vi "Generic command handler.vi"(8 "error in (no error)":errorcluster, 10 "Message in":refnum<class "GenericMessage.lvclass">, 11 "StageSPIM in":refnum<class "StageSPIM.lvclass">) -> (0 "error out":errorcluster, 2 "value":string, 3 "StageSPIM out":refnum<class "StageSPIM.lvclass">)   [LabVIEW 2012, in "StageSPIM.lvclass"]
doc: "The generic_command_handler processes the command 'generic'. Commands which are not part of the predefined list of commands fall under the 'generic' command for special activity."
uses:
  StageSPIM.lvclass
  <vilib>/Distrio/Murmex/Murmex/Murmex.lvclass
  <vilib>/Distrio/Murmex/Message/Message.lvclass
  <vilib>/Distrio/Murmex/ProceedMessage/ProceedMessage.lvclass
  <vilib>/Distrio/Murmex/GenericMessage/GenericMessage.lvclass
panel:
  # "This method is called when the GENERIC\ntrigger is sent. \n\nOverride this method when your component needs to\nrespond to this trigger. \n\nCall parent for proper implementation"
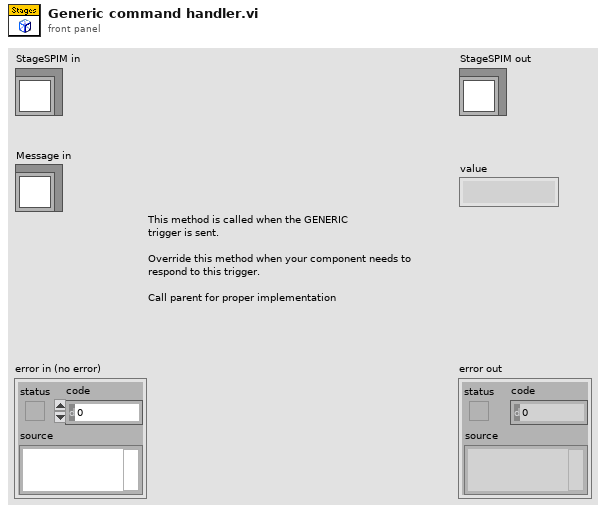
[diagram p1: front panel]
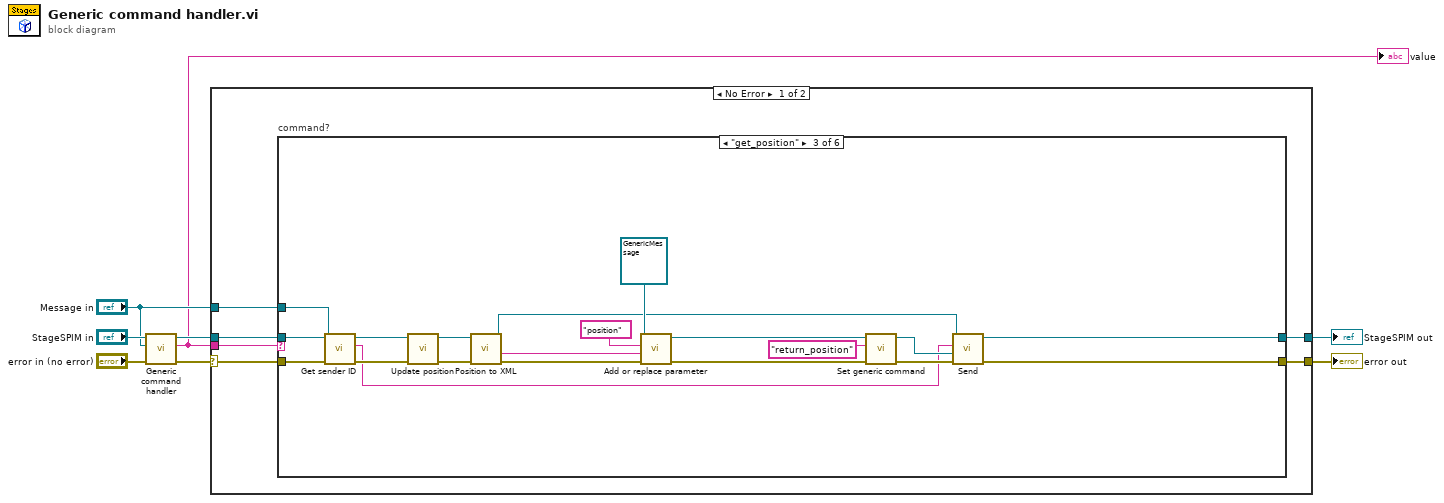
[diagram p0: block diagram]
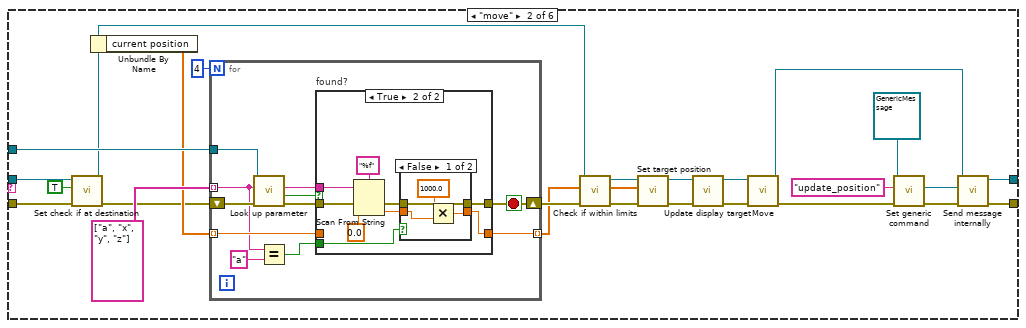
[diagram p3: hidden frame]
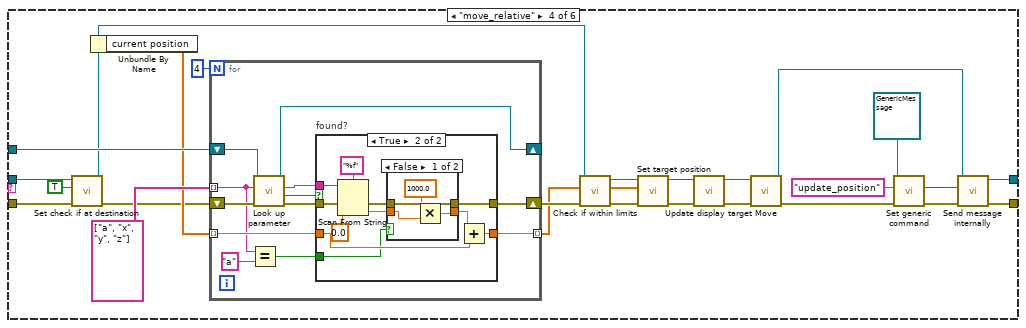
[diagram p6: hidden frame]
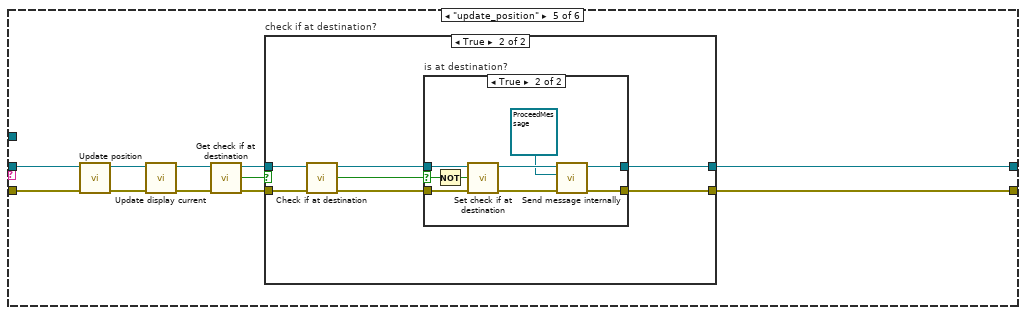
[diagram p9: hidden frame]
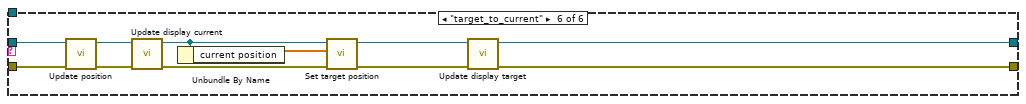
[diagram p12: hidden frame]
diagram:
  n1 = call-parent "Generic command handler.vi"("error in (no error)"="error in (no error)", "Message in"="Message in", "Murmex in"="StageSPIM in") -> ("error out"=w6:errorcluster, "value"=w3:string, "Murmex out"=w5:refnum<class "StageSPIM.lvclass">)  [unwired: 6 in]
  "value" <- w3
  n2 = case shown="No Error" w6 {
    selector: w6 -> [w13 w189]
    tunnel: w3 -> [w14 _]
    tunnel: w5 -> [w12 w190]
    tunnel: "Message in" -> [w11 _]
    tunnel: [w10 w189] -> w2
    tunnel: [w9 w190] -> w1
    frame No Error {
      n3 = case "command?" shown="\"get_position\"" w14 {
        tunnel: w13 -> [w15 w31 w89 w104 w157 w186]
        tunnel: w12 -> [w16 w33 w75 w106 w156 w185]
        tunnel: w11 -> [_ w38 w88 w111 _ _]
        tunnel: [w15 w24 w71 w97 w151 w180] -> w10
        tunnel: [w16 w21 w72 w94 w152 w178] -> w9
        frame Default {
        }
        frame "move" {
          n4 = call-dynamic "Set check if at destination.vi"("error in (no error)"=w31, "check if at destination"=TRUE, "StageSPIM in"=w33) -> ("error out"=w30:errorcluster, "StageSPIM out"=w32:refnum<class "StageSPIM.lvclass">)  [unwired: 7 in]
          n5 = Unbundle By Name(w32) -> ("current position"=w35:dbl[])
          n6 = for {
            N: 4 -> [_]
            shift-right: [w46] -> w39
            shift-left: w30 -> [w53]
            tunnel: string[] ["a", "x", "y", "z"] -> [w44] mode=indexing
            tunnel: w35 -> [w48] mode=indexing
            tunnel: [w47] -> w34 mode=indexing
            tunnel: w38 -> [w49]
            stop <- w46 stop-if-true
            n7 = call <vilib>:"Look up parameter.vi"("error in (no error)"=w53, "name"=w44, "Message in"=w49) -> ("error out"=w52:errorcluster, "found?"=w51:bool, "key"=w50:string)  [unwired: 5 in, 1 out]
            n8 = Equal?(x=w44, y="a") -> (x = y?=w43:bool)
            n9 = case "found?" shown="True" w51 {
              tunnel: w52 -> [w55 w64]
              tunnel: [w55 w59] -> w46
              tunnel: w50 -> [_ w62]
              tunnel: [w54 w57] -> w47
              tunnel: w48 -> [w54 _]
              tunnel: w43 -> [_ w56]
              frame False {
              }
              frame True {
                n10 = Scan From String(format string="%f", input string=w62, error in=w64, default 1=0.0 ("default value 1")) -> (error out=w60:errorcluster, output 1=w58:dbl)  [unwired: 1 in, 2 out]
                n11 = case shown="False" w56 {
                  tunnel: [w68 w70] -> w59
                  tunnel: w60 -> [w68 w70]
                  tunnel: [w67 w69] -> w57
                  tunnel: w58 -> [w66 w69]
                  frame False {
                    n12 = Multiply(x=1000.0, y=w66) -> (x*y=w67:dbl)
                  }
                  frame True {
                  }
                }
              }
            }
          }
          n13 = call-dynamic "Check if within limits.vi"("error in (no error)"=w39, "Position array in"=w34, "StageSPIM in"=w32) -> ("error out"=w41:errorcluster, "Approved postion array"=w40:dbl[], "StageSPIM out"=w42:refnum<class "StageSPIM.lvclass">)  [unwired: 4 in, 2 out]
          n14 = call-dynamic "Set target position.vi"("error in (no error)"=w41, "target position"=w40, "StageSPIM in"=w42) -> ("error out"=w20:errorcluster, "StageSPIM out"=w18:refnum<class "StageSPIM.lvclass">)  [unwired: 7 in]
          n15 = call-dynamic "Update display target.vi"("error in (no error)"=w20, "StageSPIM in"=w18) -> ("error out"=w19:errorcluster, "StageSPIM out"=w17:refnum<class "StageSPIM.lvclass">)  [unwired: 8 in]
          n16 = call-dynamic "Move.vi"("error in (no error)"=w19, "StageSPIM in"=w17) -> ("error out"=w28:errorcluster, "StageSPIM out"=w22:refnum<class "StageSPIM.lvclass">)  [unwired: 8 in]
          n17 = call <vilib>:"Set generic command.vi"("error in (no error)"=w28, "generic command"="update_position", "GenericMessage in"=refnum<class "GenericMessage.lvclass"> refnum ("Distrio Murmex 1.1:GenericMessage")) -> ("error out"=w27:errorcluster, "GenericMessage out"=w23:refnum<class "GenericMessage.lvclass">)  [unwired: 7 in]
          n18 = call <vilib>:"Send message internally.vi"("error in (no error)"=w27, "Message"=w23, "Murmex in"=w22) -> ("error out"=w24:errorcluster, "Murmex out"=w21:refnum<class "StageSPIM.lvclass">)  [unwired: 7 in]
        }
        frame "get_position" {
          n19 = call <vilib>:"Get sender ID.vi"("error in (no error)"=w89, "Message in"=w88) -> ("error out"=w87:errorcluster, "sender"=w83:string)  [unwired: 7 in, 1 out]
          n20 = call-dynamic "Update position.vi"("error in (no error)"=w87, "StageSPIM in"=w75) -> ("error out"=w77:errorcluster, "StageSPIM out"=w74:refnum<class "StageSPIM.lvclass">)  [unwired: 8 in]
          n21 = call-dynamic "Position to XML.vi"("error in (no error)"=w77, "StageSPIM in"=w74) -> ("error out"=w76:errorcluster, "XML string"=w73:string, "StageSPIM out"=w78:refnum<class "StageSPIM.lvclass">)  [unwired: 7 in]
          n22 = call <vilib>:"Add or replace parameter.vi"("error in (no error)"=w76, "value"=w73, "name"="position", "Message in"=refnum<class "GenericMessage.lvclass"> refnum ("Distrio Murmex 1.1:GenericMessage")) -> ("error out"=w81:errorcluster, "Message out"=w80:refnum<class "GenericMessage.lvclass">)  [unwired: 6 in]
          n23 = call <vilib>:"Set generic command.vi"("error in (no error)"=w81, "generic command"="return_position", "GenericMessage in"=w80) -> ("error out"=w85:errorcluster, "GenericMessage out"=w84:refnum<class "GenericMessage.lvclass">)  [unwired: 7 in]
          n24 = call <vilib>:"Send.vi"("error in (no error)"=w85, "Message"=w84, "recipient"=w83, "Murmex in"=w78) -> ("error out"=w71:errorcluster, "Murmex out"=w72:refnum<class "StageSPIM.lvclass">)  [unwired: 6 in]
        }
        frame "move_relative" {
          n25 = call-dynamic "Set check if at destination.vi"("error in (no error)"=w104, "check if at destination"=TRUE, "StageSPIM in"=w106) -> ("error out"=w103:errorcluster, "StageSPIM out"=w105:refnum<class "StageSPIM.lvclass">)  [unwired: 7 in]
          n26 = Unbundle By Name(w105) -> ("current position"=w108:dbl[])
          n27 = for {
            N: 4 -> [_]
            shift-right: [w124] -> w112
            shift-left: w103 -> [w127]
            tunnel: string[] ["a", "x", "y", "z"] -> [w118] mode=indexing
            shift-right: [w121] -> _
            shift-left: w111 -> [w122]
            tunnel: w108 -> [w120] mode=indexing
            tunnel: [w119] -> w107 mode=indexing
            n28 = Equal?(x=w118, y="a") -> (x = y?=w116:bool)
            n29 = call <vilib>:"Look up parameter.vi"("error in (no error)"=w127, "name"=w118, "Message in"=w122) -> ("error out"=w126:errorcluster, "found?"=w125:bool, "key"=w123:string, "Message out"=w121:refnum<class "GenericMessage.lvclass">)  [unwired: 5 in]
            n30 = case "found?" shown="True" w125 {
              tunnel: w126 -> [w129 w140]
              tunnel: [w129 w133] -> w124
              tunnel: w123 -> [_ w138]
              tunnel: [w128 w136] -> w119
              tunnel: w120 -> [w128 w135]
              tunnel: w116 -> [_ w134]
              frame False {
              }
              frame True {
                n31 = Scan From String(format string="%f", input string=w138, error in=w140, default 1=0.0 ("default value 1")) -> (error out=w132:errorcluster, output 1=w130:dbl)  [unwired: 1 in, 2 out]
                n32 = case shown="False" w134 {
                  tunnel: [w144 w146] -> w133
                  tunnel: w132 -> [w144 w146]
                  tunnel: [w143 w145] -> w131
                  tunnel: w130 -> [w142 w145]
                  frame False {
                    n33 = Multiply(x=1000.0, y=w142) -> (x*y=w143:dbl)
                  }
                  frame True {
                  }
                }
                n34 = Add(x=w131, y=w135) -> (x+y=w136:dbl)
              }
            }
          }
          n35 = call-dynamic "Check if within limits.vi"("error in (no error)"=w112, "Position array in"=w107, "StageSPIM in"=w105) -> ("error out"=w114:errorcluster, "Approved postion array"=w113:dbl[], "StageSPIM out"=w115:refnum<class "StageSPIM.lvclass">)  [unwired: 4 in, 2 out]
          n36 = call-dynamic "Set target position.vi"("error in (no error)"=w114, "target position"=w113, "StageSPIM in"=w115) -> ("error out"=w93:errorcluster, "StageSPIM out"=w90:refnum<class "StageSPIM.lvclass">)  [unwired: 7 in]
          n37 = call-dynamic "Update display target.vi"("error in (no error)"=w93, "StageSPIM in"=w90) -> ("error out"=w92:errorcluster, "StageSPIM out"=w91:refnum<class "StageSPIM.lvclass">)  [unwired: 8 in]
          n38 = call-dynamic "Move.vi"("error in (no error)"=w92, "StageSPIM in"=w91) -> ("error out"=w101:errorcluster, "StageSPIM out"=w95:refnum<class "StageSPIM.lvclass">)  [unwired: 8 in]
          n39 = call <vilib>:"Set generic command.vi"("error in (no error)"=w101, "generic command"="update_position", "GenericMessage in"=refnum<class "GenericMessage.lvclass"> refnum ("Distrio Murmex 1.1:GenericMessage")) -> ("error out"=w100:errorcluster, "GenericMessage out"=w96:refnum<class "GenericMessage.lvclass">)  [unwired: 7 in]
          n40 = call <vilib>:"Send message internally.vi"("error in (no error)"=w100, "Message"=w96, "Murmex in"=w95) -> ("error out"=w97:errorcluster, "Murmex out"=w94:refnum<class "StageSPIM.lvclass">)  [unwired: 7 in]
        }
        frame "update_position" {
          n41 = call-dynamic "Update position.vi"("error in (no error)"=w157, "StageSPIM in"=w156) -> ("error out"=w150:errorcluster, "StageSPIM out"=w148:refnum<class "StageSPIM.lvclass">)  [unwired: 8 in]
          n42 = call-dynamic "Update display current.vi"("error in (no error)"=w150, "StageSPIM in"=w148) -> ("error out"=w149:errorcluster, "StageSPIM out"=w147:refnum<class "StageSPIM.lvclass">)  [unwired: 8 in]
          n43 = call-dynamic "Get check if at destination.vi"("error in (no error)"=w149, "StageSPIM in"=w147) -> ("error out"=w154:errorcluster, "check if at destination"=w155:bool, "StageSPIM out"=w153:refnum<class "StageSPIM.lvclass">)  [unwired: 7 in]
          n44 = case "check if at destination?" shown="True" w155 {
            tunnel: w154 -> [w159 w166]
            tunnel: w153 -> [w158 w165]
            tunnel: [w158 w161] -> w152
            tunnel: [w159 w160] -> w151
            frame False {
            }
            frame True {
              n45 = call-dynamic "Check if at destination.vi"("error in (no error)"=w166, "StageSPIM in"=w165) -> ("error out"=w163:errorcluster, "at destination?"=w164:bool, "StageSPIM out"=w162:refnum<class "StageSPIM.lvclass">)  [unwired: 7 in]
              n46 = case "is at destination?" shown="True" w164 {
                selector: w164 -> [_ w176]
                tunnel: w163 -> [w168 w177]
                tunnel: w162 -> [w167 w174]
                tunnel: [w168 w170] -> w160
                tunnel: [w167 w169] -> w161
                frame False {
                }
                frame True {
                  n47 = Not(x=w176) -> (.not. x?=w175:bool)
                  n48 = call-dynamic "Set check if at destination.vi"("error in (no error)"=w177, "check if at destination"=w175, "StageSPIM in"=w174) -> ("error out"=w173:errorcluster, "StageSPIM out"=w172:refnum<class "StageSPIM.lvclass">)  [unwired: 7 in]
                  n49 = call <vilib>:"Send message internally.vi"("error in (no error)"=w173, "Message"=refnum<class "ProceedMessage.lvclass"> refnum ("Distrio Murmex 1.1:ProceedMessage"), "Murmex in"=w172) -> ("error out"=w170:errorcluster, "Murmex out"=w169:refnum<class "StageSPIM.lvclass">)  [unwired: 7 in]
                }
              }
            }
          }
        }
        frame "target_to_current" {
          n50 = call-dynamic "Update position.vi"("error in (no error)"=w186, "StageSPIM in"=w185) -> ("error out"=w188:errorcluster, "StageSPIM out"=w187:refnum<class "StageSPIM.lvclass">)  [unwired: 8 in]
          n51 = call-dynamic "Update display current.vi"("error in (no error)"=w188, "StageSPIM in"=w187) -> ("error out"=w183:errorcluster, "StageSPIM out"=w184:refnum<class "StageSPIM.lvclass">)  [unwired: 8 in]
          n52 = Unbundle By Name(w184) -> ("current position"=w182:dbl[])
          n53 = call-dynamic "Set target position.vi"("error in (no error)"=w183, "target position"=w182, "StageSPIM in"=w184) -> ("error out"=w181:errorcluster, "StageSPIM out"=w179:refnum<class "StageSPIM.lvclass">)  [unwired: 7 in]
          n54 = call-dynamic "Update display target.vi"("error in (no error)"=w181, "StageSPIM in"=w179) -> ("error out"=w180:errorcluster, "StageSPIM out"=w178:refnum<class "StageSPIM.lvclass">)  [unwired: 8 in]
        }
      }
    }
    frame Error {
    }
  }
  "error out" <- w2
  "StageSPIM out" <- w1
